vi "SCM2 Field Read.vi"(1 "Calibration":T1, 2 "Keithley GPIB Address":refnum<visa-resource-name>) -> (0 "SCM2 Field":dbl=1.0 format="%.4f")   [LabVIEW 2024]
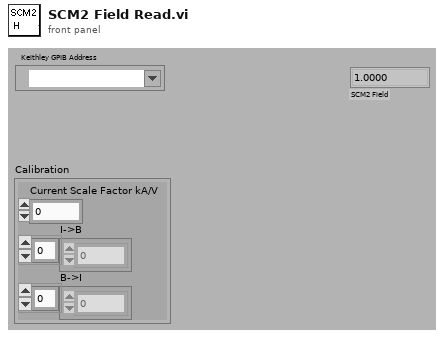
[diagram p1: front panel]
types:
  T1 = cluster{"Current Scale Factor kA/V":dbl, "I->B":dbl[], "B->I":dbl[]}
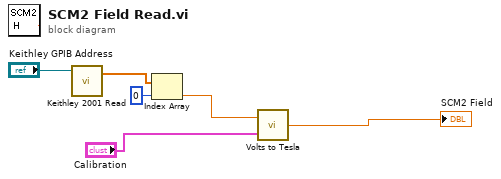
[diagram p0: block diagram]
diagram:
  n1 = call "Keithley 2001 Read.vi"("Instrument Address"="Keithley GPIB Address") -> ("Measurement"=w6:dbl[])  [unwired: 1 in, 1 out]
  n2 = Index Array(array=w6, index=0) -> (element=w4:dbl)
  n3 = call "Volts to Tesla.vi"("Calibration"="Calibration", "Console voltage"=w4) -> ("Field"=→"SCM2 Field":dbl)
